vi "流程启动命令.vi"(8 "error in (no error)":errorcluster caption="错误输入（无错误）", 10 "流程":enum16{"润洗", "进样", "加标", "搅拌", "排液"}(ring), 11 "参数":enum16{"氨氮", "总磷", "总氮", "CODMn", "CODcr"}(ring)) -> (0 "error out":errorcluster caption="错误输出")   [LabVIEW 2016, in "质控单元.lvlib"]
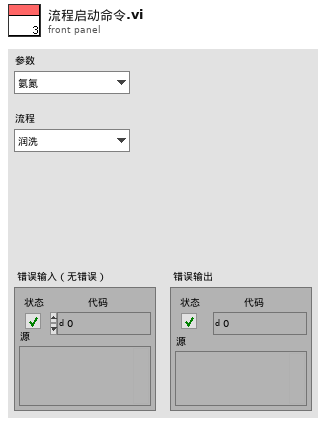
[diagram p1: front panel]
types:
  T1 = cluster{"氨氮":u8, "总磷":u8, "总氮":u8, "CODMn":u8, "CODCr":u8}
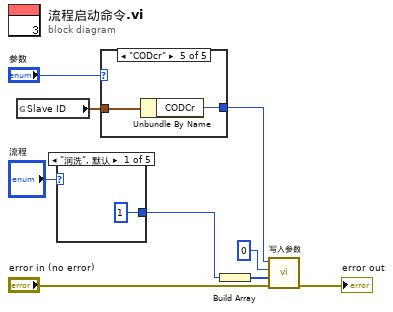
[diagram p0: block diagram]
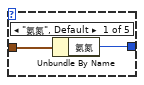
[diagram p2: hidden frame]
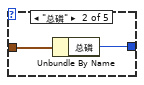
[diagram p3: hidden frame]
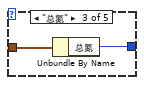
[diagram p4: hidden frame]
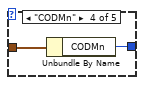
[diagram p5: hidden frame]
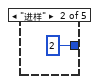
[diagram p6: hidden frame]
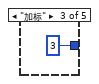
[diagram p7: hidden frame]
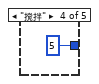
[diagram p8: hidden frame]
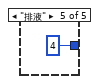
[diagram p9: hidden frame]
diagram:
  n1 = global read "断电保存全局.vi" "Slave ID"() -> (w2:T1)
  n2 = case shown="\"润洗\", 默认" "流程" {
    tunnel: [u16 1 ("quantity") u16 2 ("quantity") u16 3 ("quantity") u16 5 ("quantity") u16 4 ("quantity")] -> w5
    frame "润洗", Default {
    }
    frame "进样" {
    }
    frame "加标" {
    }
    frame "搅拌" {
    }
    frame "排液" {
    }
  }
  n3 = case shown="\"CODcr\"" "参数" {
    tunnel: w2 -> [w16 w18 w20 w22 w24]
    tunnel: [w15 w17 w19 w21 w23] -> w1
    frame "氨氮", Default {
      n4 = Unbundle By Name(w16) -> ("氨氮"=w15:u8)
    }
    frame "总磷" {
      n5 = Unbundle By Name(w18) -> ("总磷"=w17:u8)
    }
    frame "总氮" {
      n6 = Unbundle By Name(w20) -> ("总氮"=w19:u8)
    }
    frame "CODMn" {
      n7 = Unbundle By Name(w22) -> ("CODMn"=w21:u8)
    }
    frame "CODcr" {
      n8 = Unbundle By Name(w24) -> ("CODCr"=w23:u8)
    }
  }
  n9 = Build Array(w5) -> (w4:u16[])
  n10 = call "写入参数.vi"("Error in"="error in (no error)", "values"=w4, "starting address"=u16 0, "Slave ID"=w1) -> ("error out"=→"error out":errorcluster)  [unwired: 7 in]
